vi "PFI-28000-Chan-28144-V_Set Bridge Configuration.vi"(8 "error in (no error)":errorcluster, 10 "Bridge Configuration":T1, 11 "PFI-28000-Chan-28144-V in":refnum<class "PFI-28000-Chan-28144-V.lvclass">) -> (0 "error out":errorcluster, 3 "PFI-28000-Chan-28144-V out":refnum<class "PFI-28000-Chan-28144-V.lvclass">)   [LabVIEW 2017, in "PFI-28000-Chan-28144-V.lvclass"]
uses:
  PFI-28000-Chan-28144-V.lvclass
  C:/wc/07143 Precision Filters 28000 Support/Driver/source/Channel/PFI-28000-Channel.lvclass
  PFI-28000-Chan-28144-V-Bridge Configuration.ctl
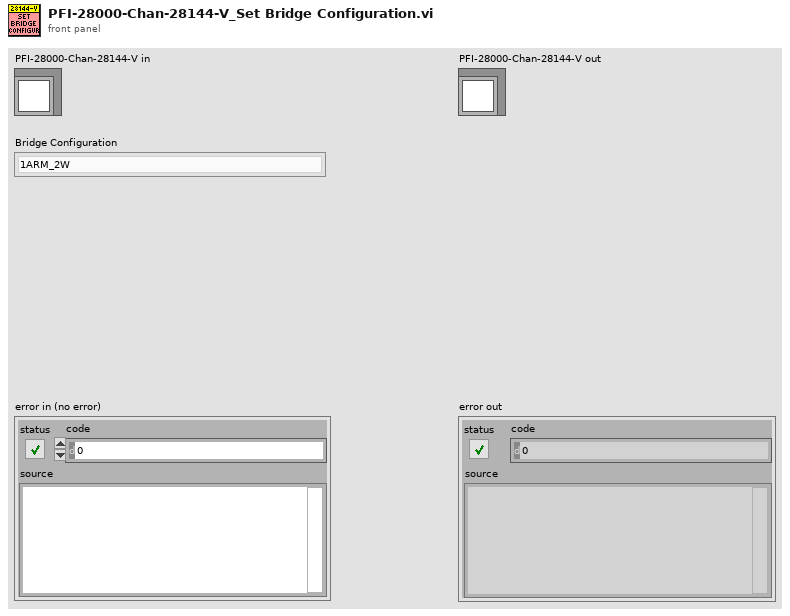
[diagram p1: front panel]
types:
  T1 = typedef "PFI-28000-Chan-28144-V.lvclass/PFI-28000-Chan-28144-V-Bridge Configuration.ctl" = enum8{"1ARM_2W", "1ARM_3W", "2ARM", "4ARM"}
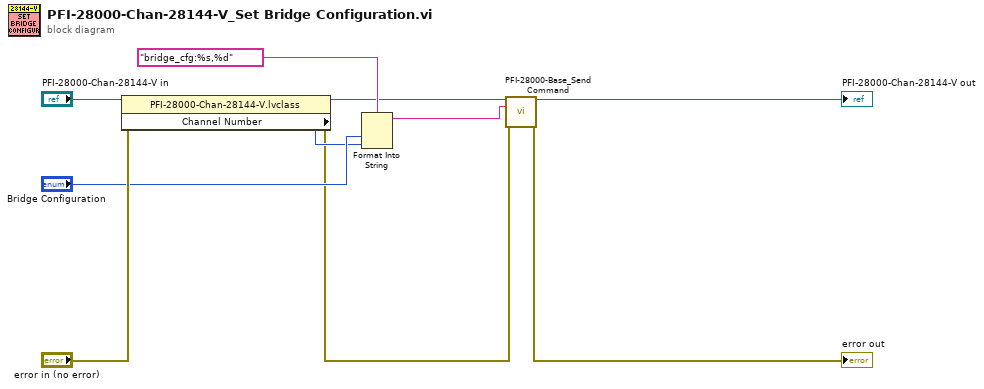
[diagram p0: block diagram]
diagram:
  n1 = property class="PFI-28000-Chan-28144-V.lvclass"(reference="PFI-28000-Chan-28144-V in", error in="error in (no error)") -> (reference out=w5:refnum<class "PFI-28000-Chan-28144-V.lvclass">, error out=w2:errorcluster, "Channel Number"=w6:i32)
  n2 = Format Into String(format string="bridge_cfg:%s,%d" ("empty string"), "Bridge Configuration", w6) -> (resulting string=w3:string)  [unwired: 2 in, 1 out]
  n3 = call-dynamic "PFI-28000-Base_Send Command.vi"("PFI-28000-Base in"=w5, "Command"=w3, "error in (no error)"=w2) -> ("PFI-28000-Base out"=→"PFI-28000-Chan-28144-V out":refnum<class "PFI-28000-Chan-28144-V.lvclass">, "error out"=→"error out":errorcluster)  [unwired: 11 in]
